vi "Read or Write Data.vi"(8 "error in":errorcluster, 10 "file exists?":bool, 11 "Path Out":path) -> (0 "error out":errorcluster, 3 "User Details":T1(array[cluster]))   [LabVIEW 2018]
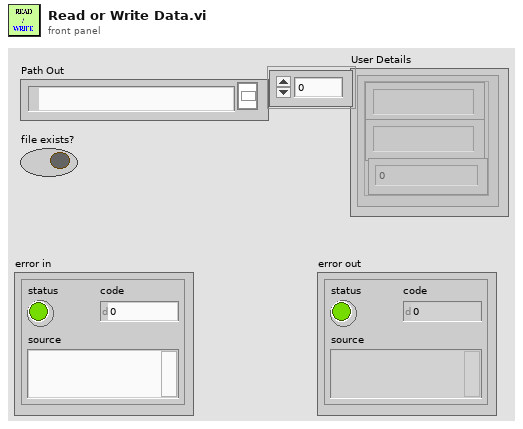
[diagram p1: front panel]
types:
  T1 = cluster{"Default User ":string, "Default Password":string, "Default User Type":u16}[]
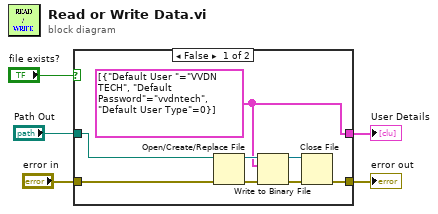
[diagram p0: block diagram]
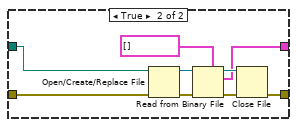
[diagram p2: hidden frame]
diagram:
  n1 = case shown="False" "file exists?" {
    tunnel: "Path Out" -> [w8 w18]
    tunnel: "error in" -> [w9 w17]
    tunnel: [w7 w16] -> w2
    tunnel: [w6 w14] -> w1
    frame False {
      w6 = T1 [{"Default User "="VVDN TECH", "Default Password"="vvdntech", "Default User Type"=0}] ("User Details")
      n2 = Open/Create/Replace File(file path (use dialog)=w8, error in=w9) -> (refnum out=w10:refnum<file>, error out=w13:errorcluster)  [unwired: 4 in, 1 out]
      n3 = Write to Binary File(file (use dialog)=w10, data=w6, error in=w13) -> (refnum out=w11:refnum<file>, error out=w12:errorcluster)  [unwired: 3 in, 1 out]
      n4 = Close File(refnum=w11, error in=w12) -> (error out=w7:errorcluster)  [unwired: 1 out]
    }
    frame True {
      n5 = Open/Create/Replace File(file path (use dialog)=w18, error in=w17) -> (refnum out=w19:refnum<file>, error out=w22:errorcluster)  [unwired: 4 in, 1 out]
      n6 = Read from Binary File(5:T1 [] ("User Details"), 8:w22, 11:w19) -> (0:w21:errorcluster, 2:w14:T1, 3:w20:refnum<file>)  [unwired: 3 in, 1 out]
      n7 = Close File(refnum=w20, error in=w21) -> (error out=w16:errorcluster)  [unwired: 1 out]
    }
  }
  "error out" <- w2
  "User Details" <- w1
